vi "LEBITVacuum.MKSreadout.vi"(7 "command":string="pz", 8 "Binary Address":u32=51, 10 "Resource Name":refnum<visa-resource-name>="COM13") -> (0 "error out":errorcluster={"status"=TRUE, "code"=-1073807339, "source"="VISA Read in LEBITVacuum.MKSreadout.vi->LEBITVacuum.lvlib:LEBITVacuum.ProcPeriodic.vi:1->BaseProcess.lvlib:BaseProcess.call proc periodic.vi:3->BaseProcess.threads 10.vi"}, 3 "Array":string[](array[string])=["$0PZ"])   [LabVIEW 2014, in "LEBITVacuum.lvlib"]
doc: "When parameters are chosen properly, this guy can read out presures from five channels."
uses:
  LEBITVacuum.lvlib
  <vilib>/Instr/_visa.llb/VISA Configure Serial Port (Instr).vi
panel:
  in  "error in (no error)":errorcluster
  # "(mb)"
  # "Channel 1"
  # "Channel 2"
  # "Channel 3"
  # "Channel 4"
  # "Channel 5"
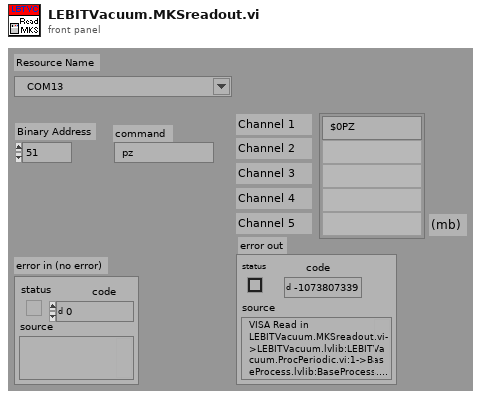
[diagram p1: front panel]
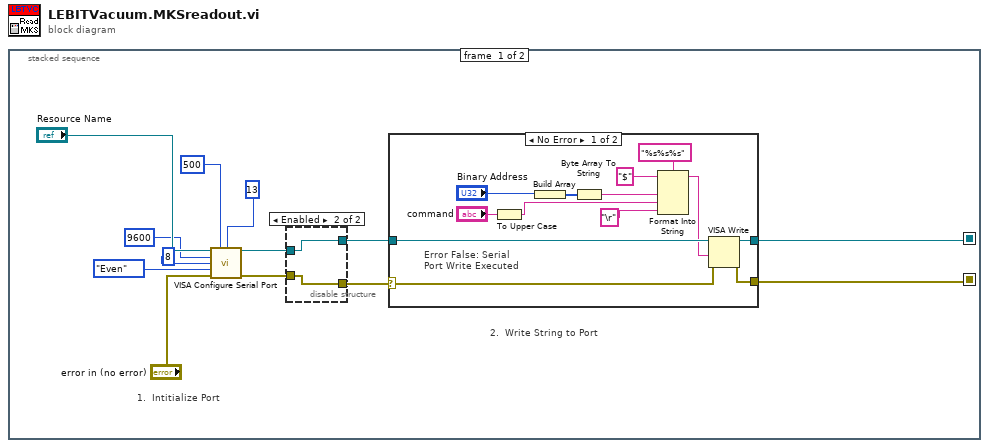
[diagram p0: block diagram]
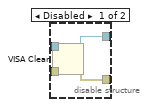
[diagram p2: hidden frame]
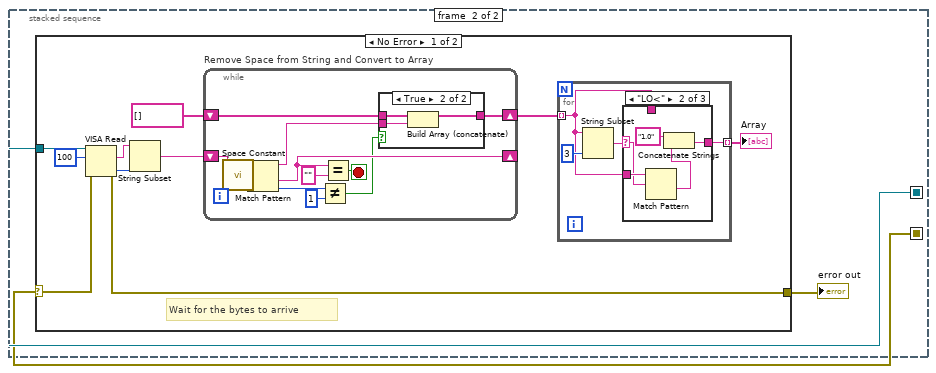
[diagram p4: hidden frame]
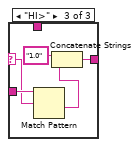
[diagram p7: hidden frame]
diagram:
  n1 = stacked-sequence {
    seq-local: [w11 _] -> [_ w37]
    seq-local: [w10 _] -> [_ w36]
    frame #0 {
      # "2.  Write String to Port"
      # "1.  Intitialize Port"
      n2 = call-poly "VISA Configure Serial Port"("VISA resource name"="Resource Name", "timeout (10sec)"=u32 500 ("Read Timeout"), "termination char\n(0xA = '\\n' = LF)"=u8 13, "baud rate (9600)"=u32 9600, "data bits (8)"=u16 8, "parity (0:none)"=enum16{"None", "Odd", "Even", "Mark", "Space"}."Even", "error in (no error)"="error in (no error)") -> ("VISA resource name out"=w9:refnum<visa-resource-name>, "error out"=w7:errorcluster)  [unwired: 7 in]
      n3 = disable-structure shown="Enabled" {
        disable-tunnel: w9 -> [w17 w19]
        disable-tunnel: [w16 w19] -> w8
        disable-tunnel: w7 -> [w15 w18]
        disable-tunnel: [w14 w18] -> w6
        frame Disabled {
          n4 = VISA Clear(VISA resource name=w17, error in (no error)=w15) -> (VISA resource name out=w16:refnum<visa-resource-name>, error out=w14:errorcluster)
        }
        frame Enabled {
        }
      }
      n5 = case shown="No Error" w6 {
        selector: w6 -> [w31 w33]
        tunnel: w8 -> [w32 w34]
        tunnel: [w30 w33] -> w10
        tunnel: [w29 w34] -> w11
        frame No Error {
          # "Error False: Serial\nPort Write Executed"
          n6 = To Upper Case(1:"command") -> (0:w23:string)
          n7 = Build Array("Binary Address") -> (w26:u32[])
          n8 = Byte Array To String(unsigned byte array=w26) -> (string=w24:string)
          n9 = Format Into String(format string="%s%s%s", initial string="$", w24, w23, "\r") -> (resulting string=w20:string)  [unwired: 1 in, 1 out]
          n10 = VISA Write(VISA resource name=w32, write buffer=w20, error in (no error)=w31) -> (VISA resource name out=w29:refnum<visa-resource-name>, error out=w30:errorcluster)  [unwired: 1 out]
        }
        frame Error {
        }
      }
    }
    frame #1 {
      n11 = case shown="No Error" w36 {
        selector: w36 -> [w45 w78]
        tunnel: [w43 w78] -> w35
        tunnel: w37 -> [w46 _]
        frame No Error {
          # "Wait for the bytes to arrive"
          n12 = VISA Read(VISA resource name=w46, byte count=u32 100 ("byte count (0)"), error in (no error)=w45) -> (read buffer=w44:string, return count=w41:u32, error out=w43:errorcluster)  [unwired: 1 out]
          n13 = String Subset(string=w44, length (rest)=w41) -> (substring=w40:string)  [unwired: 1 in]
          n14 = while "Remove Space from String and Convert to Array" {
            shift-right: [w53] -> _
            shift-left: w40 -> [w58]
            shift-right: [w55] -> w38
            shift-left: string[] [] -> [w56]
            stop <- w54 stop-if-true
            n15 = call <vilib>:"Space Constant.vi"() -> ("String"=w57:string)
            n16 = Match Pattern(string=w58, regular expression=w57) -> (before substring=w51:string, after substring=w53:string, offset past match=w50:i32)  [unwired: 1 in, 1 out]
            n17 = Not Equal?(x=w50, y=1) -> (x != y?=w48:bool)
            n18 = Equal?(x=w53, y="") -> (x = y?=w54:bool)
            n19 = case shown="True" w48 {
              tunnel: w56 -> [w59 w62]
              tunnel: [w59 w61] -> w55
              tunnel: w51 -> [_ w60]
              frame False {
              }
              frame True {
                n20 = Build Array (concatenate)(w62, w60) -> (w61:string[])
              }
            }
          }
          n21 = for {
            tunnel: w38 -> [w63] mode=indexing
            tunnel: [w64] -> w42 mode=indexing
            n22 = String Subset(string=w63, length (rest)=3 ("length (rest)")) -> (substring=w65:string)  [unwired: 1 in]
            n23 = case shown="\"LO<\"" w65 {
              selector: w65 -> [_ w69 w76]
              tunnel: [w67 w68 w75] -> w64
              tunnel: w63 -> [_ w70 w77]
              tunnel: w63 -> [w67 _ _]
              frame "False", Default {
              }
              frame "LO<" {
                n24 = Match Pattern(string=w70, regular expression=w69) -> (after substring=w71:string)  [unwired: 1 in, 3 out]
                n25 = Concatenate Strings("1.0", w71) -> (w68:string)
              }
              frame "HI>" {
                n26 = Match Pattern(string=w77, regular expression=w76) -> (after substring=w73:string)  [unwired: 1 in, 3 out]
                n27 = Concatenate Strings("1.0", w73) -> (w75:string)
              }
            }
          }
          "Array" <- w42
        }
        frame Error {
        }
      }
      "error out" <- w35
    }
  }
